vi "CCSA RPJ SLJC PR002 SubVI003.vi"(0 "Distancia d":dbl=10.0, 1 "appended array":u16[][](array[numeric])) -> (2 "Objeto rojo":dbl, 3 "Objeto verde":dbl, 4 "Objeto azul":dbl)   [LabVIEW 2021]
doc: "Algoritmo de cálculo de la distancia Z apartir de los centroides. Recibe una matriz de [2x3] y entrega 3 valores, corresondiente a tres objetos, rojo, verde y azul."
panel:
  # "CUEVAS CERÓN SERGIO ALBERTO\nREYES PÉREZ JAVIER\nSALCEDO LICEA JUAN CARLOS"
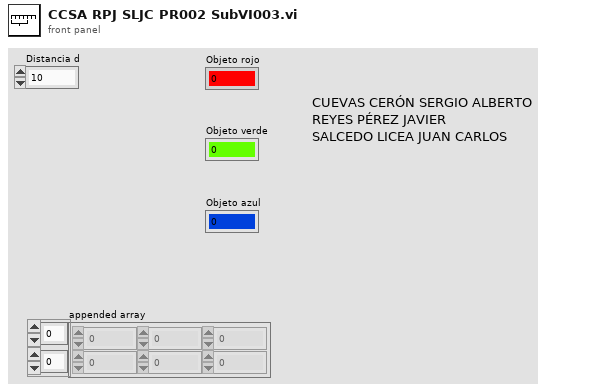
[diagram p1: front panel]
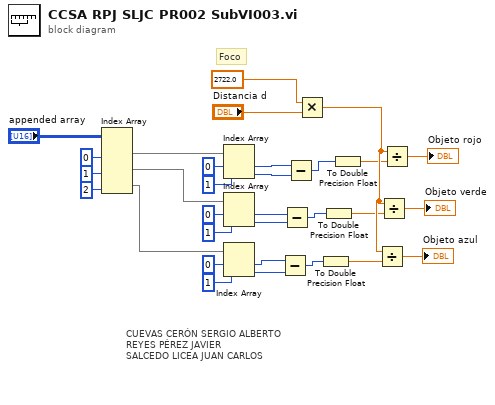
[diagram p0: block diagram]
diagram:
  # "CUEVAS CERÓN SERGIO ALBERTO\nREYES PÉREZ JAVIER\nSALCEDO LICEA JUAN CARLOS"
  # "Foco"
  n1 = Index Array(array="appended array", index (col) #1=0 ("disabled index (col)"), index (col) #2=1 ("index (col)"), index (col) #3=2 ("index (col)")) -> (element #1=w9:u16[], element #2=w10:u16[], element #3=w11:u16[])  [unwired: 3 in]
  n2 = Index Array(array=w9, index #1=0 ("index"), index #2=1 ("index")) -> (element #1=w21:u16, element #2=w22:u16)
  n3 = Index Array(array=w10, index #1=0 ("index"), index #2=1 ("index")) -> (element #1=w25:u16, element #2=w26:u16)
  n4 = Index Array(array=w11, index #1=0 ("index"), index #2=1 ("index")) -> (element #1=w29:u16, element #2=w30:u16)
  n5 = Subtract(x=w29, y=w30) -> (x-y=w28:u16)
  n6 = Subtract(x=w25, y=w26) -> (x-y=w23:u16)
  n7 = Subtract(x=w21, y=w22) -> (x-y=w4:u16)
  n8 = Multiply(x=2722.0 ("index"), y="Distancia d") -> (x*y=w31:dbl)
  n9 = To Double Precision Float(number=w28) -> (double precision float=w1:dbl)
  n10 = To Double Precision Float(number=w23) -> (double precision float=w2:dbl)
  n11 = To Double Precision Float(number=w4) -> (double precision float=w3:dbl)
  n12 = Divide(x=w31, y=w1) -> (x/y=→"Objeto azul":dbl)
  n13 = Divide(x=w31, y=w2) -> (x/y=→"Objeto verde":dbl)
  n14 = Divide(x=w31, y=w3) -> (x/y=→"Objeto rojo":dbl)
